vi "Double FFT Mesurament Test with Background Noise Remove.vi"() -> ()   [LabVIEW 2014]
uses:
  <vilib>/Platform/TimedLoop/XDataNode/timing_clust.ctl
  <vilib>/Platform/TimedLoop/XDataNode/nitl_modes.ctl
  <vilib>/Platform/TimedLoop/XDataNode/wakeup.ctl
  <vilib>/rvi/Analysis/measure/FFT/simModelSupport/niFPGA FFT Streaming Sim Properties.ctl
  <vilib>/rvi/Analysis/measure/FFT/simModelSupport/niFPGA FFT Sim Stream Group Properties.ctl
  <vilib>/rvi/Analysis/measure/FFT/simModelSupport/niFPGA FFT Sim Types.ctl
  <vilib>/rvi/Analysis/measure/FFT/simModelSupport/niFpgaFFTSimArithmeticProperties.ctl
  <vilib>/rvi/Analysis/measure/FFT/simModelSupport/niFpgaFFTSimDfxp.ctl
  <vilib>/fxp/LVFixedPointQuantizationPolicyTypeDef.ctl
  <vilib>/rvi/Analysis/measure/FFT/XNode/niFpgaFFTButterflyDelays.ctl
  <vilib>/rvi/Emulation/niFpgaSctlEmulationGetInTimedLoop.vi
  <vilib>/rvi/Emulation/niFpgaEmulationReportErrorSimple.vi
  <vilib>/rvi/Emulation/niFpgaGetClockAttributes.vi
  <vilib>/rvi/Emulation/niFpgaCriticalErrorInLSC.vi
  <vilib>/rvi/Emulation/niFpgaEmulationIsFPGAContextNoSignature.vi
  <vilib>/rvi/DataTransferAndStorage/Container/Common/niFpgaContainerGetUniqueNameForEmu.vi
  <vilib>/rvi/Memory/Memory_Emulation/niFpgaMemoryEmulationCacheClearOnFirstRun.vi
  <vilib>/rvi/Memory/Memory_Emulation/nirvimemoryEmulationManagerCache_MakeExclusive.vi
  <vilib>/rvi/Memory/Memory_Emulation/niFpgaMemoryEmulationValidateCache.vi
  <vilib>/rvi/Memory/Memory_Emulation/nirvimemoryEmulationManagerCache_InsertValue.vi
  <vilib>/Utility/error.llb/Clear Errors.vi
  <vilib>/rvi/Memory/Memory_Emulation/nirvimemoryEmulationManagerCache_ReleaseExclusive.vi
  <vilib>/rvi/Memory/Memory_Emulation/nirvimemoryEmulationManagerCache_GetValue.vi
  <vilib>/rvi/Memory/Memory_Emulation/nirvimemoryEmulationManagerCache_SetValue.vi
  <vilib>/rvi/Emulation/niFpgaProcessEmulError.vi
  <vilib>/rvi/errors/niFpgaSetErrorForExecOnDevCompSimple.vi
  <vilib>/rvi/eio/common/nirviEmuReportErrorAndStop.vi
  <vilib>/rvi/FIFO/Fifo_Resource/nirvififoEmulationSetSize.vi
  <vilib>/rvi/FIFO/Fifo_Resource/nirviFifoEmulationQueueMgr.vi
  <instcachedir>/0/nirviFifoEmulationQueueMgr_E5CAEC123FF24DC58D834DCA3CDAA9B5.lvgen/nirviFifoEmulationQueueMgr_E5CAEC123FF24DC58D834DCA3CDAA9B5_010.vi
  <vilib>/rvi/FIFO/Fifo_Resource/nirvififoEmulationCreateLock.vi
  <vilib>/rvi/FIFO/Fifo_Resource/nirvififoEmulationObtainLock.vi
  <vilib>/rvi/FIFO/Fifo_Resource/nirvififoEmulationReleaseLock.vi
  <vilib>/rvi/occurrence/nirviWaitOnOccurrenceBase.vi
  <vilib>/rvi/errors/nirviReportUnexpectedCaseInternalError.vi
  <vilib>/rvi/errors/nirviReportUnexpectedCaseInternalError (U32).vi
  <vilib>/rvi/FIFO/Fifo_Resource/nirvififoEmulationDetermineInputValidOut.vi
  <vilib>/rvi/Memory/Memory_Emulation/nirvimemoryFastEmulation.vi
  <vilib>/rvi/Memory/Memory_Emulation/nirvimemoryEmulation.vi
  <vilib>/rvi/Analysis/measure/FFT/simModelSupport/niFpgaFFTSimModelStreamingCore.vi
  <vilib>/rvi/interface/RandomDataEmulation/niFpgaRandomDataHandleErrors.vi
  <vilib>/rvi/eio/common/nirviEmuTemplateMethod_errors.vi
  <vilib>/Platform/TimedLoop/XDataNode/XDataNode.xnode
  <vilib>/rvi/DataTransferAndStorage/Container/XNode/niFpgaContainer.xnode
  <vilib>/rvi/DataTransferAndStorage/Register/Emulation/niFpgaRegisterEmulation.vi
  <vilib>/rvi/FIFO/Fifo_Resource/nirvififoEmulationRead.vi
  <vilib>/rvi/FIFO/Fifo_Resource/nirvififoEmulationWrite.vi
  <vilib>/rvi/Analysis/measure/FFT/XNode/niFpgaFFT.xnode
  <vilib>/rvi/interface/RandomDataEmulation/nirviRandomDataFpgaReadWriteTemplate.vi
  <vilib>/eio/EIOMethodNode/EIOMethodNode.xnode
  <vilib>/Platform/TimedLoop/XDataNode/XDNodeRunTimeDep.lvlib
panel:
  in  "n-bit (2^nbit medie)":i32=8
  in  "Latency points":u32
  in  "snapshot":bool
  in  "lower limit 2":u32=682
  in  "lower limit 1":u32=57
  in  "upper limit 2":u32=1193
  in  "upper limit 1":u32=568
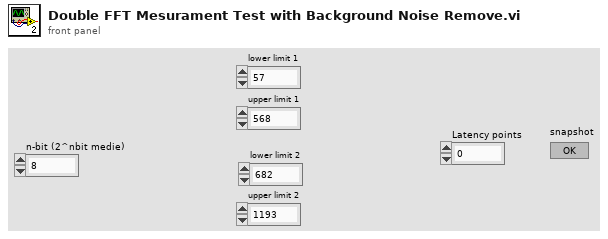
[diagram p1: front panel]
types:
  T1 = typedef "XDNodeRunTimeDep.lvlib/timing_clust.ctl" = cluster{"Expected End [f-1]":u64, "Actual End [f-1]":u64, "Finished Late? [f-1]":bool, "Expected End [i-1]":u64, "Actual End [i-1]":u64, "Finished Late? [i-1]":bool, "Expected Start [i]":u64, "Actual Start [i]":u64, "Expected Start [f]":u64, "Actual Start [f]":u64, "Source Name":string, "Structure Name":string, "Period":i64, "Deadline":i64, "Offset":i64, "Start":i64, "Priority":i32, "Timeout":i32, "Mode":T2, "Wakeup Reason":T3, "Error":errorcluster, "Source Type":string, "Secondary Source Type":string, "Global End Time":u64, "Global Start Time":u64, "Frame Duration":u64, "Iteration Duration":u64, "Assigned CPU":i32, "I/O Scan Engine Mode":u32}
  T2 = typedef "XDNodeRunTimeDep.lvlib/nitl_modes.ctl" = enum32{"No Change", "Process missed periods, maintain original phase", "Discard missed periods, maintain original phase", "Process missed periods, ignore original phase", "Discard missed periods, ignore original phase"}
  T3 = typedef "XDNodeRunTimeDep.lvlib/wakeup.ctl" = enum32{"Normal", "Aborted", "Asynchronous wakeup", "Timing source error", "Timed loop error", "Timeout"}
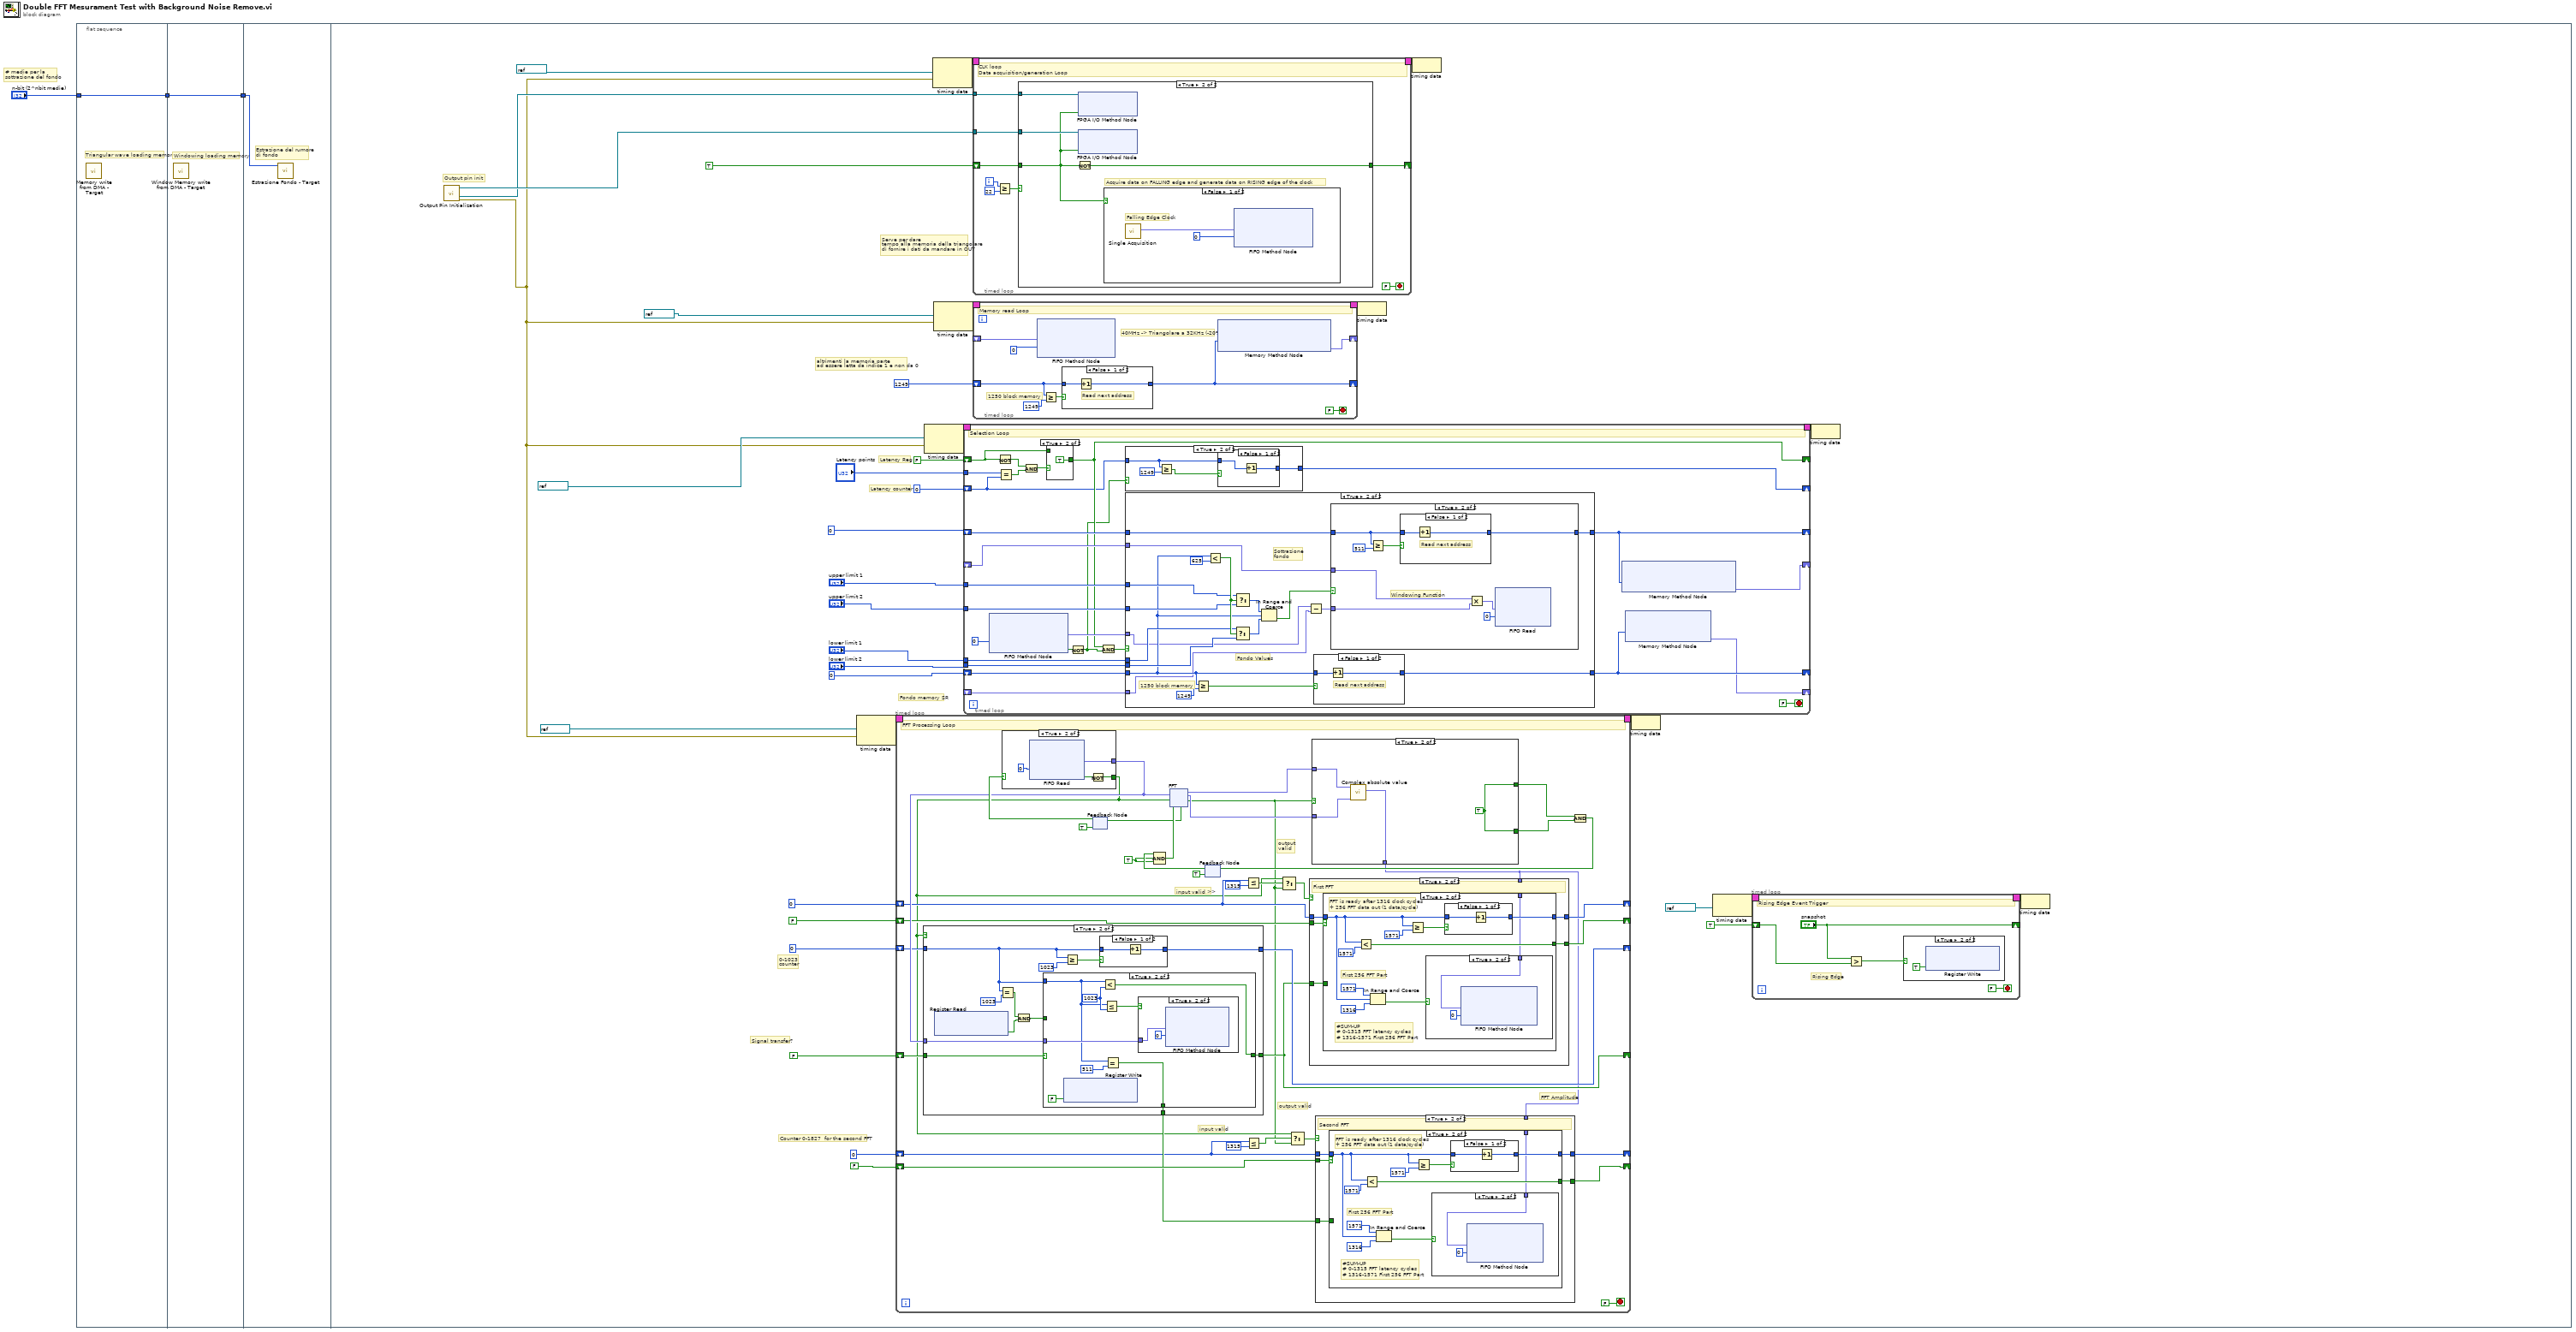
[diagram p0: block diagram]
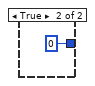
[diagram p4: hidden frame]
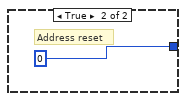
[diagram p8: hidden frame]
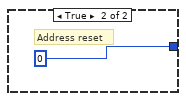
[diagram p9: hidden frame]
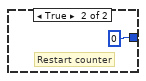
[diagram p13: hidden frame]
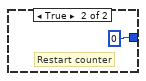
[diagram p17: hidden frame]
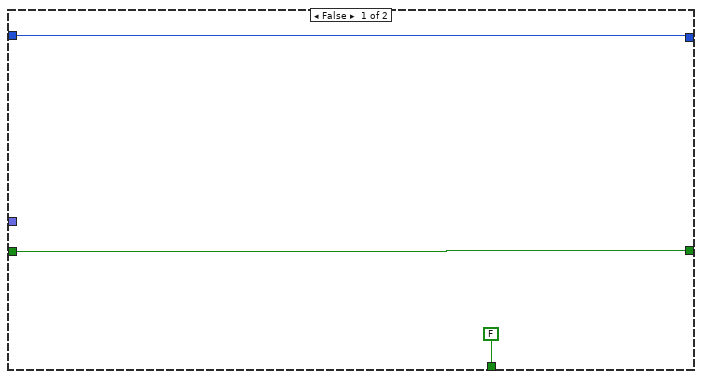
[diagram p18: hidden frame]
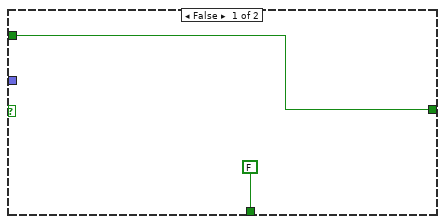
[diagram p19: hidden frame]
diagram:
  # "# medie per la\nsottrazione del fondo"
  n1 = flat-sequence {
    tunnel: [w4] -> w3
    tunnel: "n-bit (2^nbit medie)" -> [w4]
    tunnel: w3 -> [w5]
    tunnel: [w5] -> w1
    tunnel: w1 -> [w6]
    frame #0 {
      # "Triangular wave loading memory"
      n2 = call "Memory write from DMA - Target.vi"() -> ()  [unwired: 12 in]
    }
    frame #1 {
      # "Windowing loading memory"
      n3 = call "Window Memory write from DMA - Target.vi"() -> ()  [unwired: 12 in]
    }
    frame #2 {
      # "Estrazione del rumore\ndi fondo"
      n4 = call "Estrazione Fondo - Target.vi"("n-bit (2^nbit medie)"=w6) -> ()  [unwired: 11 in]
    }
    frame #3 {
      # "Fondo memory SR"
      # "altrimenti la memoria parte \nad essere letta da indice 1 e non da 0"
      # "Serve per dare\ntempo alla memoria della triangolare\ndi fornire i dati da mandare in OUT"
      # "Latency counter"
      # "Latency Reg"
      # "Counter 0-1827  for the second FFT"
      # "0-1023\ncounter"
      # "Signal transfer?"
      # "Output pin init"
      n5 = call "Output Pin Initialization.vi"() -> ("error out"=w25:errorcluster, "I/O Out Clock DAC (pin16)"=w29:refnum<k21>, "I/O Out Clock ADC (pin17)"=w30:refnum<k21>)  [unwired: 8 in]
      n6 = node-c288(refnum<k21> "40MHz" ("Source Name"), w25) -> (w38:T1)
      n7 = timed-loop {
        timing: w38 -> [_]
        timing-out: [_] -> w37
        shift-right: [w152] -> _
        shift-left: FALSE -> [w155]
        shift-right: [w156] -> _
        shift-left: i16 0 -> [w153]
        shift-right: [w151] -> _
        shift-left: FALSE -> [w150]
        shift-right: [w149] -> _
        shift-left: i16 0 -> [w147]
        shift-right: [w144] -> _
        shift-left: i16 0 -> [w137]
        shift-right: [w141] -> _
        shift-left: FALSE -> [w142]
        stop <- FALSE stop-if-true
        w133 = TRUE
        # "output valid"
        # "input valid"
        # "FFT Amplitude"
        # "output\nvalid"
        # "input valid >>"
        # "FFT Processing Loop"
        n8 = feedback #1(TRUE ("ready for input")) -> (w168:bool)
        n9 = case shown="True" w168 {
          tunnel: [FALSE w285] -> w136
          tunnel: [fxp<+/-,12,12> 0.0 ("Element") w282] -> w154
          frame False {
            # "RMS is not ready for new input"
          }
          frame True {
            n10 = xnode ("FIFO Read")("Timeout"=0) -> ("Element"=w282:fxp<+/-,12,12>, "Timed Out?"=w284:bool)  [unwired: 1 in, 1 out]
            n11 = Not(x=w284) -> (.not. x?=w285:bool)
          }
        }
        n12 = case shown="True" w136 {
          tunnel: w153 -> [w221 w227]
          tunnel: [w221 w231] -> w156
          tunnel: w155 -> [w220 w225]
          tunnel: [w220 w226] -> w152
          tunnel: w154 -> [_ w224]
          tunnel: [FALSE w222] -> w140
          frame False {
          }
          frame True {
            n13 = xnode ("Register Read")() -> ("Data"=w223:bool)  [unwired: 1 in, 1 out]
            n14 = Equal?(x=w227, y=i16 1023) -> (x = y?=w230:bool)
            n15 = And(x=w230, y=w223) -> (x .and. y?=w228:bool)
            n16 = case shown="True" w225 {
              tunnel: w228 -> [w235 _]
              tunnel: w227 -> [_ w238]
              tunnel: [w235 w243] -> w226
              tunnel: w224 -> [_ w241]
              tunnel: [FALSE w236] -> w222
              frame False {
              }
              frame True {
                w240 = i16 1023 ("y")
                n17 = xnode ("Register Write")("Data"=FALSE) -> ()  [unwired: 1 in, 1 out]
                n18 = Less?(x=w238, y=w240) -> (x < y?=w243:bool)
                n19 = Less Or Equal?(x=w238, y=w240) -> (x <= y?=w242:bool)
                n20 = Equal?(x=w238, y=i16 511) -> (x = y?=w236:bool)
                n21 = case shown="True" w242 {
                  tunnel: w241 -> [_ w244]
                  frame False {
                  }
                  frame True {
                    n22 = xnode ("FIFO Method Node")("Element"=w244, "Timeout"=0) -> ()  [unwired: 1 in, 2 out]
                  }
                }
              }
            }
            n23 = Greater Or Equal?(x=w227, y=i16 1023) -> (x >= y?=w232:bool)
            n24 = case shown="False" w232 {
              tunnel: w227 -> [w247 _]
              tunnel: [w246 i16 0] -> w231
              frame False {
                n25 = Increment(x=w247) -> (x+1=w246:i16)
              }
              frame True {
                # "Restart counter"
              }
            }
          }
        }
        n26 = feedback #2(TRUE) -> (w164:bool)
        n27 = Compound Arithmetic op=AND(w164, w133, w133) -> (w163:bool)
        n28 = xnode "FFT"("real data in"=w154, "input valid"=w136, "ready for output"=w163) -> ("ready for input"=w162:bool, "real data out"=w161:fxp<+/-,22,22>, "imaginary data out"=w160:fxp<+/-,22,22>, "output valid"=w134:bool)  [unwired: 2 in, 1 out]
        n29 = feedback-in #1(w162) -> ()
        n30 = Less Or Equal?(x=w147, y=i16 1315) -> (x <= y?=w148:bool)
        n31 = Less Or Equal?(x=w137, y=i16 1315) -> (x <= y?=w138:bool)
        n32 = Select(t=w136, s=w148, f=w134) -> (s? t:f=w145:bool)
        n33 = Select(t=w136, s=w138, f=w134) -> (s? t:f=w135:bool)
        n34 = case shown="True" w134 {
          tunnel: w161 -> [_ w279]
          tunnel: w160 -> [_ w278]
          tunnel: [w275 w276] -> w159
          tunnel: [w275 w276] -> w158
          tunnel: [_ w277] -> w143
          frame False {
            w275 = TRUE
          }
          frame True {
            w276 = TRUE
            n35 = call "Complex absolute value.vi"("Im"=w278, "Re"=w279) -> ("Square Absolute Value"=w277:fxp<+,44,44>)  [unwired: 9 in]
          }
        }
        n36 = case shown="True" w145 {
          tunnel: w152 -> [_ w201]
          tunnel: [w194 w200] -> w151
          tunnel: w150 -> [w194 w199]
          tunnel: w147 -> [w195 w198]
          tunnel: [w195 w197] -> w149
          tunnel: w143 -> [_ w196]
          frame False {
          }
          frame True {
            # "First FFT"
            n37 = case shown="True" w199 {
              tunnel: w201 -> [w203 _]
              tunnel: [w203 w213] -> w200
              tunnel: w198 -> [w202 w206]
              tunnel: [w202 w209] -> w197
              tunnel: w196 -> [_ w204]
              frame False {
              }
              frame True {
                # "First 256 FFT Part"
                # "#SUM-UP\n# 0-1315 FFT latency cycles\n# 1316-1571 First 256 FFT Part"
                # "FFT is ready after 1316 clock cycles\n+ 256 FFT data out (1 data/cycle)"
                n38 = Less?(x=w206, y=i16 1571) -> (x < y?=w213:bool)
                n39 = In Range and Coerce(upper limit=i16 1571, x=w206, lower limit=i16 1316 ("y")) -> (In Range?=w205:bool)  [unwired: 1 out]
                n40 = Greater Or Equal?(x=w206, y=i16 1571) -> (x >= y?=w210:bool)
                n41 = case shown="True" w205 {
                  tunnel: w204 -> [_ w215]
                  frame False {
                  }
                  frame True {
                    n42 = xnode ("FIFO Method Node")("Element"=w215, "Timeout"=0) -> ()  [unwired: 1 in, 2 out]
                  }
                }
                n43 = case shown="False" w210 {
                  tunnel: w206 -> [w217 _]
                  tunnel: [w216 i16 0] -> w209
                  frame False {
                    n44 = Increment(x=w217) -> (x+1=w216:i16)
                  }
                  frame True {
                    # "Restart counter"
                  }
                }
              }
            }
          }
        }
        n45 = case shown="True" w135 {
          tunnel: w140 -> [_ w176]
          tunnel: [w169 w175] -> w141
          tunnel: w142 -> [w169 w174]
          tunnel: w137 -> [w170 w173]
          tunnel: [w170 w172] -> w144
          tunnel: w143 -> [_ w171]
          frame False {
          }
          frame True {
            # "Second FFT"
            n46 = case shown="True" w174 {
              tunnel: w176 -> [w178 _]
              tunnel: [w178 w188] -> w175
              tunnel: w173 -> [w177 w181]
              tunnel: [w177 w184] -> w172
              tunnel: w171 -> [_ w179]
              frame False {
              }
              frame True {
                # "First 256 FFT Part"
                # "#SUM-UP\n# 0-1315 FFT latency cycles\n# 1316-1571 First 256 FFT Part"
                # "FFT is ready after 1316 clock cycles\n+ 256 FFT data out (1 data/cycle)"
                n47 = Less?(x=w181, y=i16 1571) -> (x < y?=w188:bool)
                n48 = In Range and Coerce(upper limit=i16 1571, x=w181, lower limit=i16 1316 ("y")) -> (In Range?=w180:bool)  [unwired: 1 out]
                n49 = Greater Or Equal?(x=w181, y=i16 1571) -> (x >= y?=w185:bool)
                n50 = case shown="True" w180 {
                  tunnel: w179 -> [_ w190]
                  frame False {
                  }
                  frame True {
                    n51 = xnode ("FIFO Method Node")("Element"=w190, "Timeout"=0) -> ()  [unwired: 1 in, 2 out]
                  }
                }
                n52 = case shown="False" w185 {
                  tunnel: w181 -> [w192 _]
                  tunnel: [w191 i16 0] -> w184
                  frame False {
                    n53 = Increment(x=w192) -> (x+1=w191:i16)
                  }
                  frame True {
                    # "Restart counter"
                  }
                }
              }
            }
          }
        }
        n54 = Compound Arithmetic op=AND(w159, w158) -> (w157:bool)
        n55 = feedback-in #2(w157) -> ()
      }
      n56 = node-c288(refnum<k21> "40MHz" ("Source Name"), w25) -> (w36:T1)
      n57 = node-c288(refnum<k21> "80MHz" ("Source Name"), w25) -> (w42:T1)
      n58 = node-c288(refnum<k21> "40MHz" ("Source Name"), w25) -> (w40:T1)
      n59 = timed-loop {
        timing: w36 -> [_]
        timing-out: [_] -> w35
        shift-right: [w56] -> _
        shift-left: u32 0 -> [w66]
        tunnel: "upper limit 1" -> [w75]
        tunnel: "upper limit 2" -> [w74]
        tunnel: "lower limit 1" -> [w73]
        tunnel: "lower limit 2" -> [w72]
        shift-right: [w68] -> _
        shift-left: u32 0 -> [w71]
        shift-right: [w69] -> _
        shift-left: _ -> [w70]
        shift-right: [w60] -> _
        shift-left: FALSE -> [w61]
        tunnel: "Latency points" -> [w65]
        shift-right: [w58] -> _
        shift-left: u32 0 -> [w57]
        shift-right: [w55] -> _
        shift-left: _ -> [w54]
        stop <- FALSE stop-if-true
        # "Selection Loop"
        n60 = xnode ("FIFO Method Node")("Timeout"=0) -> ("Element"=w77:fxp<+/-,12,12>, "Timed Out?"=w78:bool)  [unwired: 1 in, 1 out]
        n61 = Not(x=w61) -> (.not. x?=w64:bool)
        n62 = Equal?(x=w65, y=w57) -> (x = y?=w63:bool)
        n63 = And(x=w64, y=w63) -> (x .and. y?=w62:bool)
        n64 = case shown="True" w62 {
          tunnel: [w88 TRUE] -> w60
          tunnel: w61 -> [w88 _]
          frame False {
          }
          frame True {
          }
        }
        n65 = Not(x=w78) -> (.not. x?=w59:bool)
        n66 = And(x=w60, y=w59) -> (x .and. y?=w67:bool)
        n67 = case shown="True" w59 {
          tunnel: w57 -> [w80 w83]
          tunnel: [w80 w81] -> w58
          frame False {
          }
          frame True {
            n68 = Greater Or Equal?(x=w83, y=u32 1249) -> (x >= y?=w82:bool)
            n69 = case shown="False" w82 {
              tunnel: w83 -> [w86 _]
              tunnel: [w85 u32 0] -> w81
              frame False {
                n70 = Increment(x=w86) -> (x+1=w85:u32)
              }
              frame True {
              }
            }
          }
        }
        n71 = case shown="True" w67 {
          tunnel: [w91 w108] -> w56
          tunnel: w66 -> [w91 w95]
          tunnel: w77 -> [_ w94]
          tunnel: w75 -> [_ w103]
          tunnel: w74 -> [_ w102]
          tunnel: w73 -> [_ w101]
          tunnel: w72 -> [_ w100]
          tunnel: w71 -> [w90 w97]
          tunnel: [w90 w99] -> w68
          tunnel: w70 -> [_ w98]
          tunnel: w54 -> [_ w92]
          frame False {
          }
          frame True {
            # "Sottrazione\nfondo"
            # "Fondo Values"
            # "1250 block memory"
            n72 = Greater Or Equal?(x=w95, y=u32 1249) -> (x >= y?=w109:bool)
            n73 = Less?(x=w95, y=u32 625) -> (x < y?=w104:bool)
            n74 = Select(t=w101, s=w104, f=w100) -> (s? t:f=w106:u32)
            n75 = Select(t=w103, s=w104, f=w102) -> (s? t:f=w107:u32)
            n76 = In Range and Coerce(upper limit=w107, x=w95, lower limit=w106) -> (In Range?=w96:bool)  [unwired: 1 out]
            n77 = Subtract(x=w94, y=w92) -> (x-y=w93:fxp<+/-,12,12>)
            n78 = case shown="False" w109 {
              tunnel: w95 -> [w124 _]
              tunnel: [w123 u32 0] -> w108
              frame False {
                # "Read next address"
                n79 = Increment(x=w124) -> (x+1=w123:u32)
              }
              frame True {
                # "Address reset"
              }
            }
            n80 = case shown="True" w96 {
              tunnel: w93 -> [_ w112]
              tunnel: w97 -> [w111 w117]
              tunnel: [w111 w119] -> w99
              tunnel: w98 -> [_ w115]
              frame False {
              }
              frame True {
                # "Windowing Function"
                n81 = Greater Or Equal?(x=w117, y=u32 511) -> (x >= y?=w118:bool)
                n82 = case shown="False" w118 {
                  tunnel: w117 -> [w121 _]
                  tunnel: [w120 u32 0] -> w119
                  frame False {
                    # "Read next address"
                    n83 = Increment(x=w121) -> (x+1=w120:u32)
                  }
                  frame True {
                    # "Address reset"
                  }
                }
                n84 = Multiply(x=w115, y=w112) -> (x*y=w113:fxp<+/-,12,12>)
                n85 = xnode ("FIFO Read")("Element"=w113, "Timeout"=0) -> ()  [unwired: 1 in, 2 out]
              }
            }
          }
        }
        n86 = xnode ("Memory Method Node")("Address"=w68) -> ("Data"=w69:fxp<+,8,1>)  [unwired: 1 in, 1 out]
        n87 = xnode ("Memory Method Node")("Address"=w56) -> ("Data"=w55:fxp<+/-,12,12>)  [unwired: 1 in, 1 out]
      }
      n88 = timed-loop {
        timing: w42 -> [_]
        timing-out: [_] -> w41
        shift-right: [w316] -> _
        shift-left: TRUE -> [w314]
        tunnel: w29 -> [w318]
        tunnel: w30 -> [w315]
        i -> [w312]
        stop <- FALSE stop-if-true
        # "CLK loop\nData acquisition/generation Loop"
        n89 = Greater Or Equal?(x=w312, y=22) -> (x >= y?=w311:bool)
        n90 = case shown="True" w311 {
          tunnel: w318 -> [_ w323]
          tunnel: [w319 w322] -> w316
          tunnel: w315 -> [_ w321]
          tunnel: w314 -> [w319 w320]
          frame False {
          }
          frame True {
            # "Acquire data on FALLING edge and generate data on RISING edge of the clock"
            n91 = Not(x=w320) -> (.not. x?=w322:bool)
            n92 = xnode "FPGA I/O Method Node"("FPGA I/O In"=w323, "Data"=w320) -> ()  [unwired: 1 out]
            n93 = xnode "FPGA I/O Method Node"("FPGA I/O In"=w321, "Data"=w320) -> ()  [unwired: 1 out]
            n94 = case shown="False" w320 {
              frame False {
                # "Falling Edge Clock"
                n95 = call "Single Acquisition.vi"() -> ("Out"=w325:fxp<+/-,12,12>)  [unwired: 10 in, 1 out]
                n96 = xnode ("FIFO Method Node")("Element"=w325, "Timeout"=0) -> ()  [unwired: 1 in, 2 out]
              }
              frame True {
                # "Rising Edge Clock"
                n97 = xnode ("FIFO Method Node")("Timeout"=0) -> ("Element"=w326:fxp<+/-,12,12>, "Timed Out?"=w327:bool)  [unwired: 1 in, 1 out]
                n98 = case shown="False" w327 {
                  tunnel: w326 -> [w331 _]
                  frame False {
                    # "Data Generation"
                    n99 = Add(x=w331, y=fxp<+,12,12> 2048.0) -> (x+y=w329:fxp<+/-,14,14>)
                    n100 = call "Single Point Wave generation.vi"("Data To Write"=w329) -> ()  [unwired: 10 in, 1 out]
                  }
                  frame True {
                    # "FPGA memory slow"
                  }
                }
              }
            }
          }
        }
      }
      n101 = timed-loop {
        timing: w40 -> [_]
        timing-out: [_] -> w39
        shift-right: [w293] -> _
        shift-left: u32 1249 -> [w297]
        shift-right: [w295] -> _
        shift-left: _ -> [w294]
        stop <- FALSE stop-if-true
        # "40MHz -> Triangolare a 32KHz (-20%)"
        # "1250 block memory"
        # "Memory read Loop"
        n102 = xnode ("FIFO Method Node")("Element"=w294, "Timeout"=0) -> ()  [unwired: 1 in, 2 out]
        n103 = Greater Or Equal?(x=w297, y=u32 1249) -> (x >= y?=w299:bool)
        n104 = case shown="False" w299 {
          tunnel: w297 -> [w302 _]
          tunnel: [w301 u32 0] -> w293
          frame False {
            # "Read next address"
            n105 = Increment(x=w302) -> (x+1=w301:u32)
          }
          frame True {
            # "Address reset"
          }
        }
        n106 = xnode ("Memory Method Node")("Address"=w293) -> ("Data"=w295:fxp<+/-,12,12>)  [unwired: 1 in, 1 out]
      }
      n107 = node-c288(w39) -> ()
      n108 = node-c288(w41) -> ()
      n109 = node-c288(w37) -> ()
      n110 = node-c288(refnum<k21> "40MHz" ("Source Name")) -> (w15:T1)
      n111 = timed-loop {
        timing: w15 -> [_]
        timing-out: [_] -> w14
        shift-right: ["snapshot"] -> _
        shift-left: TRUE ("snapshot") -> [w45]
        stop <- FALSE stop-if-true
        # "Rising Edge"
        # "Rising Edge Event Trigger"
        n112 = Greater?(x="snapshot", y=w45) -> (0:w43:bool)
        n113 = case shown="True" w43 {
          frame False {
          }
          frame True {
            n114 = xnode ("Register Write")("Data"=TRUE) -> ()  [unwired: 1 in, 1 out]
          }
        }
      }
      n115 = node-c288(w35) -> ()
      n116 = node-c288(w14) -> ()
    }
  }
